vi "Kelvinox_Change_Loop_Mode.vi"(8 "error in (no error)":errorcluster, 10 "Kelvinox-Cluster":T2, 11 "Connection Details (in)":T1={"Mode"=enum."Immediate", "Bytes to Read"=5000, "IP Address"="172.25.187.107", "Remote Port"=33576, "Timeout"=10000, "connection ID"=refnum}) -> (0 "error out":errorcluster)   [LabVIEW 2019]
uses:
  Monitor Communication/Kelvinox/Kelvinox_Control.ctl
panel:
  # "Pressures in mbar"
  # "Temperatures in K"
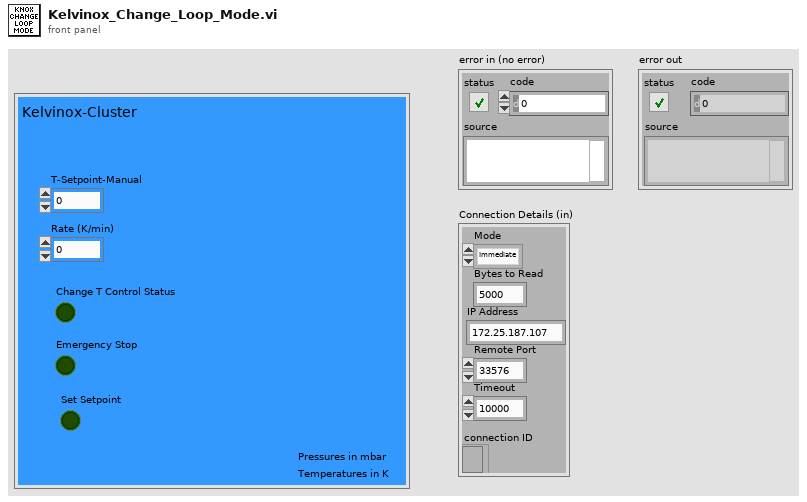
[diagram p1: front panel]
types:
  T1 = cluster{"Mode":enum16{"Standard", "Buffered", "CRLF", "Immediate"}, "Bytes to Read":i32, "IP Address":string, "Remote Port":i32, "Timeout":i32, "connection ID":refnum<k5>}
  T2 = typedef "Kelvinox_Control.ctl" = cluster{"T-Setpoint-Manual":dbl, "Rate (K/min)":dbl, "Change T Control Status":bool, "Emergency Stop":bool, "Set Setpoint":bool}
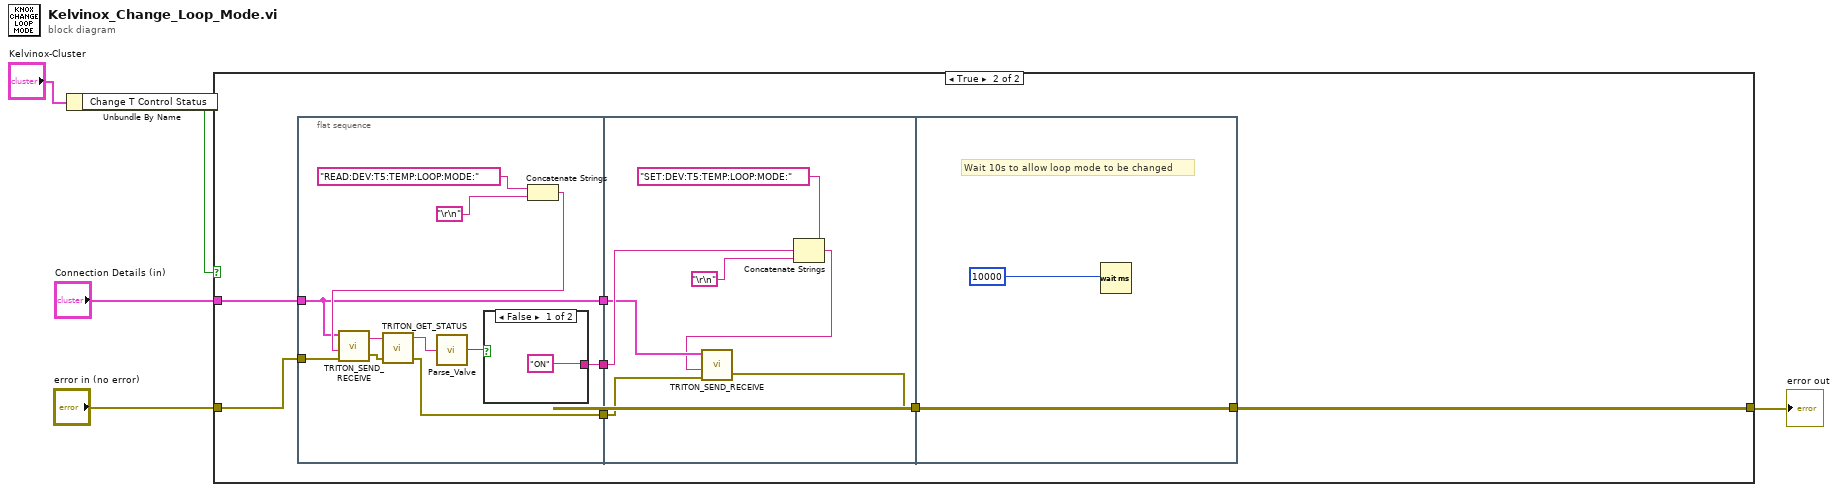
[diagram p0: block diagram]
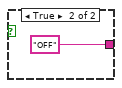
[diagram p3: hidden frame]
diagram:
  n1 = Unbundle By Name("Kelvinox-Cluster") -> ("Change T Control Status"=w4:bool)
  n2 = case shown="True" w4 {
    tunnel: "error in (no error)" -> [w6 w13]
    tunnel: [w6 w12] -> w2
    tunnel: "Connection Details (in)" -> [_ w11]
    frame False {
    }
    frame True {
      n3 = flat-sequence {
        tunnel: w13 -> [w24]
        tunnel: w11 -> [w14]
        tunnel: [w18] -> w10
        tunnel: [w17] -> w9
        tunnel: [w14] -> w8
        tunnel: w10 -> [w29]
        tunnel: w9 -> [w31]
        tunnel: w8 -> [w30]
        tunnel: [w27] -> w7
        tunnel: [w35] -> w12
        tunnel: w7 -> [w35]
        frame #0 {
          n4 = Concatenate Strings("READ:DEV:T5:TEMP:LOOP:MODE:", "\r\n") -> (w21:string)
          n5 = call "TRITON_SEND_RECEIVE.vi"("error in (no error)"=w24, "Command String"=w21, "Communication Cluster"=w14) -> ("error out"=w19:errorcluster, "Response String"=w20:string)  [unwired: 1 in]
          n6 = call "TRITON_GET_STATUS.vi"("error in (no error)"=w19, "Response String"=w20) -> ("error out"=w18:errorcluster, "Status"=w16:string)  [unwired: 2 in]
          n7 = call "Parse_Valve.vi"("Valve"=w16) -> ("Status"=w15:bool)
          n8 = case shown="False" w15 {
            tunnel: ["ON" "OFF"] -> w17
            frame False {
            }
            frame True {
            }
          }
        }
        frame #1 {
          n9 = Concatenate Strings("SET:DEV:T5:TEMP:LOOP:MODE:", w31, "\r\n") -> (w28:string)
          n10 = call "TRITON_SEND_RECEIVE.vi"("error in (no error)"=w29, "Command String"=w28, "Communication Cluster"=w30) -> ("error out"=w27:errorcluster)  [unwired: 1 in, 1 out]
        }
        frame #2 {
          # "Wait 10s to allow loop mode to be changed"
          n11 = Wait (ms)(milliseconds to wait=10000) -> ()  [unwired: 1 out]
        }
      }
    }
  }
  "error out" <- w2
